vi "XML Script - Append Terminal Name (Next Iteration).vi"(1 "loop":string) -> (0 "loop.Next Iteration":string)   [LabVIEW 2020]
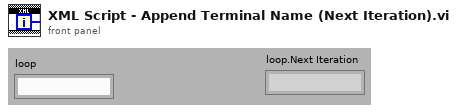
[diagram p1: front panel]
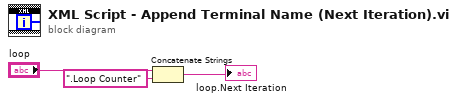
[diagram p0: block diagram]
diagram:
  n1 = Concatenate Strings("loop", ".Loop Counter" ("string")) -> (→"loop.Next Iteration":string)
